vi "EdgeUnderMouse.vi"(8 "error in (no error)":errorcluster, 9 "threshold":dbl=6.0, 10 "Coords":T1, 11 "FSM in":refnum<class "FSM.Graph.lvclass">) -> (0 "error out":errorcluster, 1 "contains mouse":bool, 2 "Edge":refnum<class "FSM.Edge.lvclass">, 3 "Edge Index":i32)   [LabVIEW 2015, in "FSM.Graph.lvclass"]
uses:
  FSM.Graph.lvclass
  <vilib>/Utility/miscctls.llb/LVPoint32TypeDef.ctl
  FSM.Edge/FSM.Edge.lvclass
  FSM.Graph.lvclass/FSM.Graph.ctl
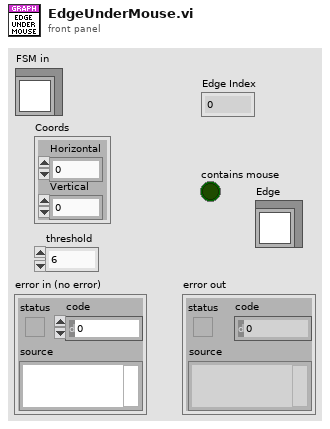
[diagram p1: front panel]
types:
  T1 = typedef "LVPoint32TypeDef.ctl" = cluster{"Horizontal":i32, "Vertical":i32}
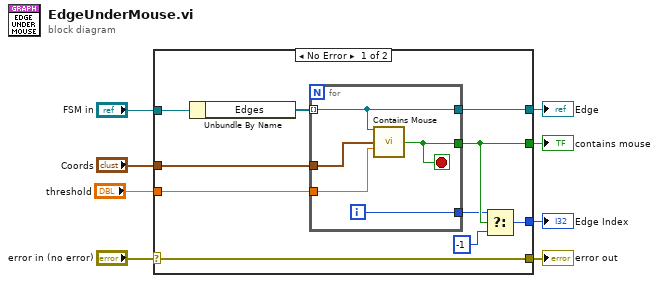
[diagram p0: block diagram]
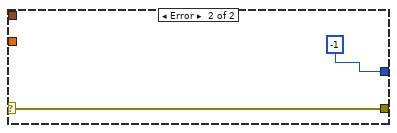
[diagram p2: hidden frame]
diagram:
  n1 = case shown="No Error" "error in (no error)" {
    selector: "error in (no error)" -> [w18 w25]
    tunnel: [w18 w25] -> w7
    tunnel: "FSM in" -> [w17 _]
    tunnel: "Coords" -> [w16 _]
    tunnel: [w13 _] -> w4
    tunnel: [w14 -1] -> w3
    tunnel: [w10 _] -> w2
    tunnel: "threshold" -> [w9 _]
    frame No Error {
      n2 = Unbundle By Name(w17) -> ("Edges"=w15:refnum<class "FSM.Edge.lvclass">[])
      n3 = for {
        tunnel: w16 -> [w21]
        tunnel: [w20] -> w13
        tunnel: w15 -> [w22] mode=indexing
        tunnel: [w23] -> w12
        tunnel: [w22] -> w10
        tunnel: w9 -> [w19]
        i -> [w23]
        stop <- w20 stop-if-true
        n4 = call "Contains Mouse.vi"("FSM.Edge"=w22, "Coords"=w21, "threshold"=w19) -> ("contains mouse"=w20:bool)  [unwired: 12 in]
      }
      n5 = Select(t=w12, s=w13, f=-1) -> (s? t:f=w14:i32)
    }
    frame Error {
    }
  }
  "error out" <- w7
  "contains mouse" <- w4
  "Edge Index" <- w3
  "Edge" <- w2
